vi "Teleop_Globals.vi"() -> ()   [LabVIEW 2019]
panel:
  out "DrivingMode":i32
  out "Joy0-POV":i32[](array[numeric])
  out "Joy0-Buttons":bool[](array[boolean])
  out "Joy0-Axes":dbl[](array[numeric])
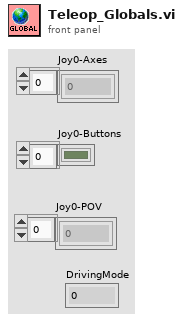
[diagram p1: front panel]
diagram:
